vi "Setup.vi"(11 "Base Queue Actor in":refnum<class "Base Queue Actor.lvclass">) -> (3 "Base Queue Actor out":refnum<class "Base Queue Actor.lvclass">)   [LabVIEW 2021, in "jettl.lvlib" / "Base Queue Actor.lvclass"]
uses:
  Base Queue Actor.lvclass
  Base Queue Actor.lvclass/Base Queue Actor.ctl
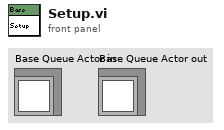
[diagram p1: front panel]
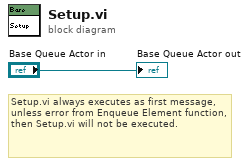
[diagram p0: block diagram]
diagram:
  # "Setup.vi always executes as first message, unless error from Enqueue Element function, then Setup.vi will not be executed."
  "Base Queue Actor out" <- "Base Queue Actor in"
